vi "平铺顺序结构.vi"() -> ()   [LabVIEW 2015]
panel:
  out "String":string
  out "随机数":dbl
  out ">= 70?":bool
  # "注意：如何修改Caption"
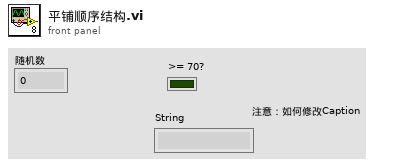
[diagram p1: front panel]
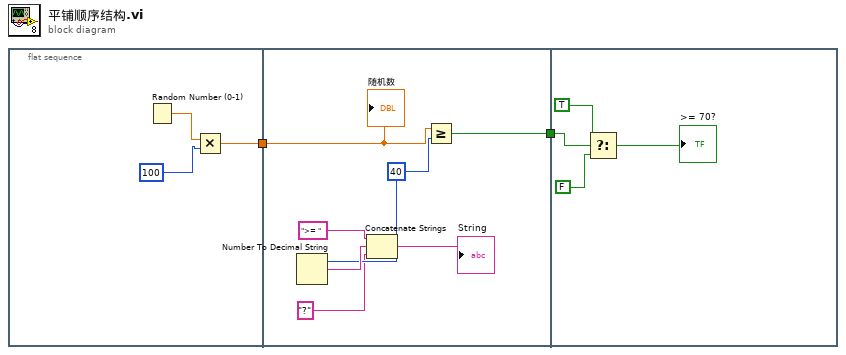
[diagram p0: block diagram]
diagram:
  n1 = flat-sequence {
    tunnel: [w3] -> w2
    tunnel: w2 -> [w11]
    tunnel: [w12] -> w1
    tunnel: w1 -> [w16]
    frame #0 {
      n2 = Random Number (0-1)() -> (number: 0 to 1=w5:dbl)
      n3 = Multiply(x=w5, y=100) -> (x*y=w3:dbl)
    }
    frame #1 {
      w8 = 40
      n4 = Number To Decimal String(number=w8) -> (decimal integer string=w9:string)  [unwired: 1 in]
      n5 = Concatenate Strings(">= ", w9, "?") -> (→"String":string)
      n6 = Greater Or Equal?(x=w11, y=w8) -> (x >= y?=w12:bool)
      "随机数" <- w11
    }
    frame #2 {
      n7 = Select(t=TRUE, s=w16, f=FALSE) -> (s? t:f=→">= 70?":bool)
    }
  }
